vi "Untitled 3.vi"() -> ()   [LabVIEW 2024]
panel:
  out "Numeric 2":u32
  in  "Numeric":u32 format="%.0x"
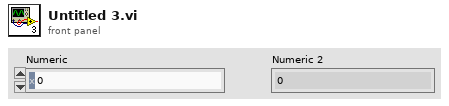
[diagram p1: front panel]
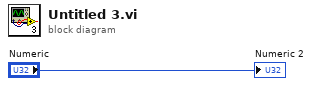
[diagram p0: block diagram]
diagram:
  "Numeric 2" <- "Numeric"
